vi "Clear RTDriver VIs.vi"(8 "error in (no error)":errorcluster, 11 "Device Item Ref in in":T1 format="%.0x") -> (0 "error out":errorcluster, 3 "Device Item Ref out":T1 format="%.0x")   [LabVIEW 2023, in "HPS-17000 Custom Device System Explorer.lvlib"]
uses:
  <vilib>/NI VeriStand/Custom Device API/Custom Device Item Ref.ctl
  NationalInstruments.VeriStand.SystemDefinitionAPI
  NationalInstruments.VeriStand.SystemStorage
  HPS-17000 Custom Device System Explorer.lvlib
  <vilib>/NI VeriStand/Custom Device API/Custom Device API.lvlib
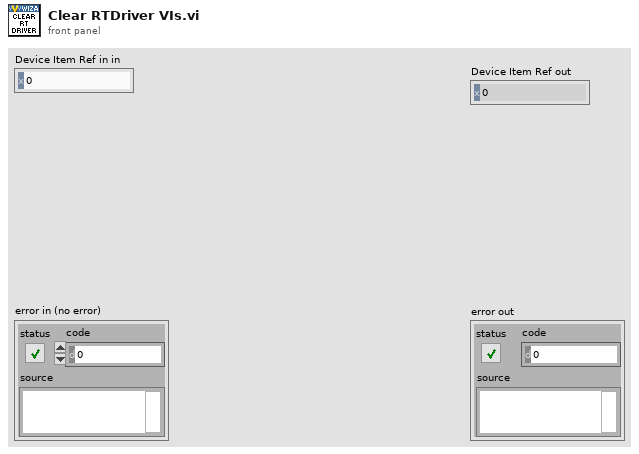
[diagram p1: front panel]
types:
  T1 = typedef "Custom Device API.lvlib/Custom Device Item Ref.ctl" = u64
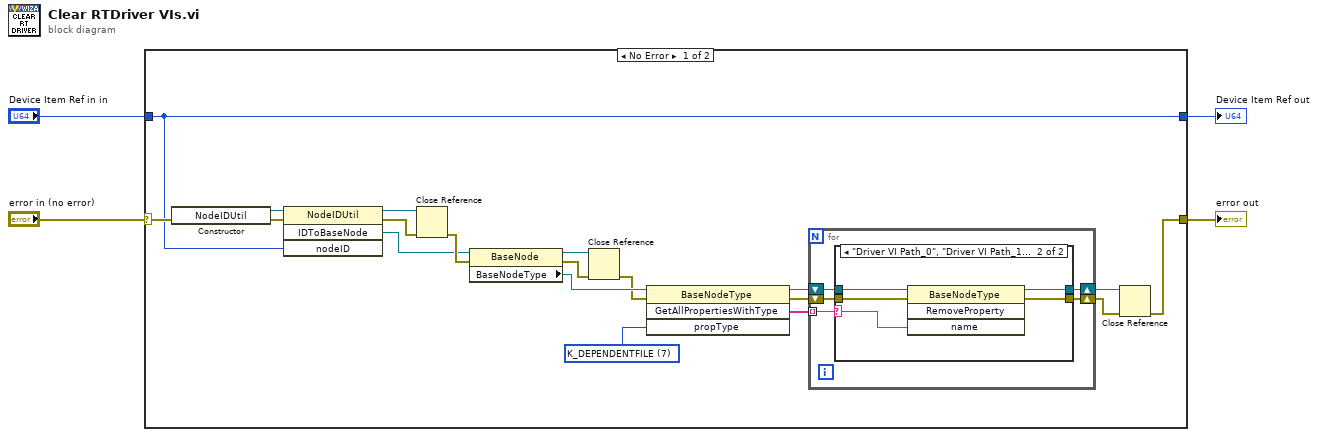
[diagram p0: block diagram]
diagram:
  n1 = case shown="No Error" "error in (no error)" {
    selector: "error in (no error)" -> [w14 w37]
    tunnel: "Device Item Ref in in" -> [w13 w36]
    tunnel: [w13 w36] -> w2
    tunnel: [w23 w37] -> w1
    frame No Error {
      w11 = 7 items=["K_STRING", "K_BOOL", "K_I32", "K_U32", "K_DOUBLE", "K_U64", "K_VARIANT", "K_DEPENDENTFILE", "K_DEPENDENTNODE", "K_DATASOURCENODE", "K_U16", "K_DBLARR", "K_U32ARR", "K_I32ARR", "K_STRINGARR", "K_DICTIONARY", "K_DICTIONARYARR", "K_BINARYSTRING", "K_I16", "K_I64", "K_BOOLARR", "K_U64ARR", "K_U16ARR", "K_I64ARR", "K_I16ARR"] ("propType")
      n2 = constructor class="NodeIDUtil"(error in=w14) -> (reference out=w15:refnum<k24>, error out=w16:errorcluster)  [unwired: 2 in, 1 out]
      n3 = invoke class="NodeIDUtil" method="IDToBaseNode"(reference=w15, error in=w16, "nodeID"=w13) -> (reference out=w20:refnum<k24>, error out=w18:errorcluster, "IDToBaseNode"=w17:refnum<k24>)  [unwired: 1 in, 1 out]
      n4 = Close Reference(reference=w20, error in (no error)=w18) -> (error out=w19:errorcluster)
      n5 = property class="BaseNode"(reference=w17, error in=w19) -> (reference out=w21:refnum<k24>, error out=w22:errorcluster, "BaseNodeType"=w8:refnum<k24>)
      n6 = Close Reference(reference=w21, error in (no error)=w22) -> (error out=w7:errorcluster)
      n7 = invoke class="BaseNodeType" method="GetAllPropertiesWithType"(reference=w8, error in=w7, "propType"=w11) -> (reference out=w10:refnum<k24>, error out=w12:errorcluster, "GetAllPropertiesWithType"=w9:string[])  [unwired: 1 in, 1 out]
      n8 = for {
        tunnel: w9 -> [w24] mode=indexing
        shift-right: [w26] -> w6
        shift-left: w12 -> [w27]
        shift-right: [w25] -> w5
        shift-left: w10 -> [w28]
        n9 = case shown="\"Driver VI Path_0\", \"Driver VI Path_1\", \"Driver VI Path_2\", \"Driver VI Path_3\", \"Driver VI Path_4\"" w24 {
          selector: w24 -> [_ w31]
          tunnel: w28 -> [w30 w35]
          tunnel: w27 -> [w29 w34]
          tunnel: [w29 w33] -> w26
          tunnel: [w30 w32] -> w25
          frame "None", Default {
          }
          frame "Driver VI Path_0", "Driver VI Path_1", "Driver VI Path_2", "Driver VI Path_3", "Driver VI Path_4" {
            n10 = invoke class="BaseNodeType" method="RemoveProperty"(reference=w35, error in=w34, "name"=w31) -> (reference out=w32:refnum<k24>, error out=w33:errorcluster)  [unwired: 1 in, 2 out]
          }
        }
      }
      n11 = Close Reference(reference=w5, error in (no error)=w6) -> (error out=w23:errorcluster)
    }
    frame Error {
    }
  }
  "Device Item Ref out" <- w2
  "error out" <- w1
